vi "_builtins_rect_map_controls.vi"(11 "MasterBndRects in":T1[][](array[typedef])) -> (1 "row_heights":i16[](array[numeric]), 2 "column_widths":i16[](array[numeric]), 3 "Resolved MasterBndRects out":T1[][](array[typedef]))   [LabVIEW 2019, in "Script.lvlib"]
doc: "Resolves the front panel control bounds using a row and column mapper.\n\nCreated by: Ryan Pacini"
uses:
  Script.lvlib
  <vilib>/Utility/miscctls.llb/LVRectTypeDef.ctl
  <vilib>/Utility/miscctls.llb/LVBoundsTypeDef.ctl
  <vilib>/Utility/miscctls.llb/LVPositionTypeDef.ctl
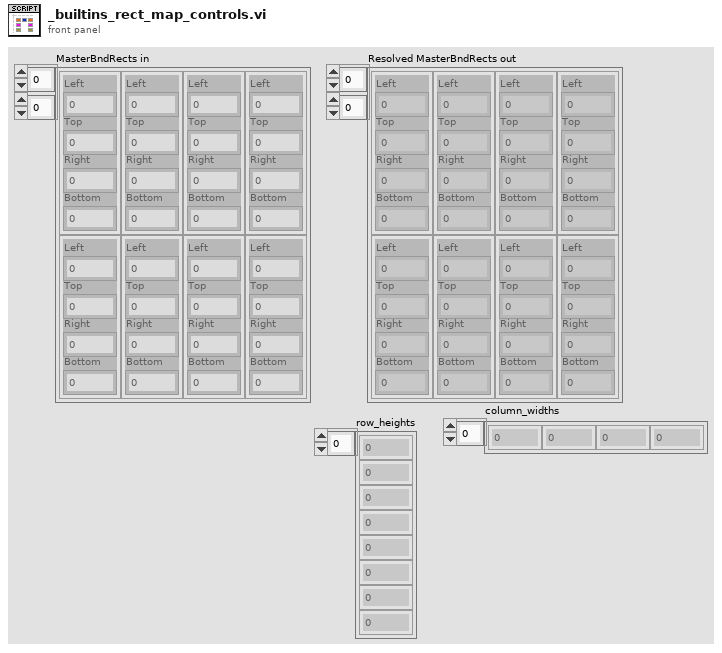
[diagram p1: front panel]
types:
  T1 = typedef "LVRectTypeDef.ctl" = cluster{"Left":i16, "Top":i16, "Right":i16, "Bottom":i16}
  T2 = typedef "LVBoundsTypeDef.ctl" = cluster{"Width":u32, "Height":u32}
  T3 = typedef "LVPositionTypeDef.ctl" = cluster{"Left":i32, "Top":i32}
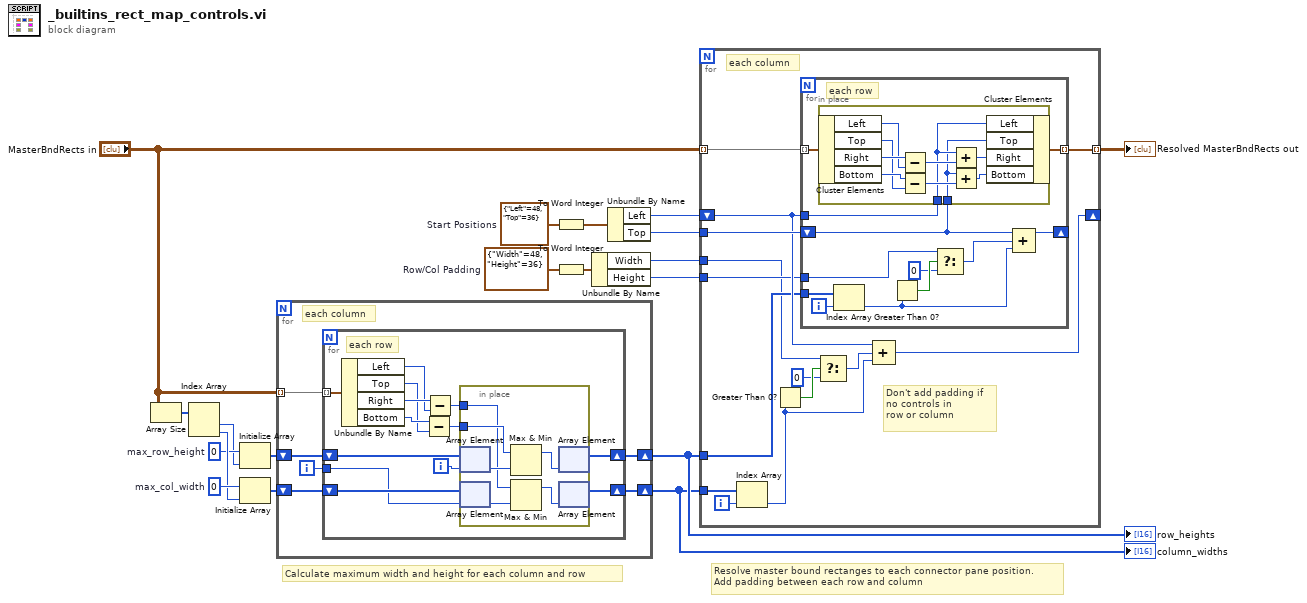
[diagram p0: block diagram]
diagram:
  w8 = i16 0  # max_row_height
  w12 = i16 0  # max_col_width
  w16 = T2 {"Width"=48, "Height"=36}  # Row/Col Padding
  w19 = T3 {"Left"=48, "Top"=36}  # Start Positions
  # "Resolve master bound rectanges to each connector pane position.\nAdd padding between each row and column"
  # "Calculate maximum width and height for each column and row"
  n1 = Array Size(array="MasterBndRects in") -> (size(s)=w11:i32[])
  n2 = Index Array(array=w11) -> (element #1=w7:i32, element #2=w9:i32)  [unwired: 2 in]
  n3 = Initialize Array(w8, w7) -> (w6:i16[])
  n4 = Initialize Array(w12, w9) -> (w4:i16[])
  n5 = for {
    tunnel: "MasterBndRects in" -> [w25] mode=indexing
    shift-right: [w23] -> w5
    shift-left: w6 -> [w24]
    shift-right: [w21] -> w3
    shift-left: w4 -> [w22]
    i -> [w20]
    # "each column"
    n6 = for {
      tunnel: w25 -> [w38] mode=indexing
      shift-right: [w29] -> w23
      shift-left: w24 -> [w33]
      shift-right: [w28] -> w21
      shift-left: w22 -> [w32]
      tunnel: w20 -> [w26]
      i -> [w27]
      # "each row"
      n7 = Unbundle By Name(w38) -> ("Left"=w35:i16, "Top"=w34:i16, "Right"=w37:i16, "Bottom"=w36:i16)
      n8 = Subtract(x=w36, y=w34) -> (x-y=w31:i16)
      n9 = Subtract(x=w37, y=w35) -> (x-y=w30:i16)
      n10 = in-place {
        in-place-border: w31 -> [w43]
        in-place-border: w30 -> [w40]
        n11 = in-place-array #1(w33, w27) -> (w44:i16)
        n12 = in-place-array #2(w32, w26) -> (w41:i16)
        n13 = Max & Min(x=w43, y=w44) -> (max(x,y)=w42:i16)  [unwired: 1 out]
        n14 = Max & Min(x=w40, y=w41) -> (max(x,y)=w39:i16)  [unwired: 1 out]
        n15 = in-place-array #1(w42) -> (w29:i16[])  [unwired: 1 out]
        n16 = in-place-array #2(w39) -> (w28:i16[])  [unwired: 1 out]
      }
    }
  }
  "row_heights" <- w5
  "column_widths" <- w3
  n17 = To Word Integer(number=w19) -> (16bit integer=w18:cluster{"Left":i16, "Top":i16})
  n18 = To Word Integer(number=w16) -> (16bit integer=w17:cluster{"Width":i16, "Height":i16})
  n19 = Unbundle By Name(w17) -> ("Width"=w2:i16, "Height"=w1:i16)
  n20 = Unbundle By Name(w18) -> ("Left"=w14:i16, "Top"=w13:i16)
  n21 = for {
    tunnel: "MasterBndRects in" -> [w57] mode=indexing
    tunnel: [w58] -> w15 mode=indexing
    tunnel: w5 -> [w52]
    shift-right: [w54] -> _
    shift-left: w14 -> [w55]
    tunnel: w13 -> [w56]
    tunnel: w3 -> [w51]
    tunnel: w2 -> [w46]
    tunnel: w1 -> [w50]
    i -> [w53]
    # "Don't add padding if\nno controls in\nrow or column"
    # "each column"
    n22 = Index Array(array=w51, index=w53) -> (element=w47:i16)
    n23 = Greater Than 0?(x=w47) -> (x > 0?=w49:bool)
    n24 = for {
      tunnel: [w70] -> w58 mode=indexing
      tunnel: w57 -> [w69] mode=indexing
      shift-right: [w68] -> _
      shift-left: w56 -> [w67]
      tunnel: w55 -> [w66]
      tunnel: w52 -> [w65]
      tunnel: w50 -> [w60]
      i -> [w64]
      # "each row"
      n25 = in-place {
        in-place-border: w67 -> [w71]
        in-place-border: w66 -> [w72]
        n26 = in-place-cluster #3(w69) -> ("Left"=w79:i16, "Top"=w77:i16, "Right"=w80:i16, "Bottom"=w78:i16)
        n27 = Subtract(x=w80, y=w79) -> (x-y=w76:i16)
        n28 = Subtract(x=w78, y=w77) -> (x-y=w74:i16)
        n29 = Add(x=w72, y=w76) -> (x+y=w75:i16)
        n30 = Add(x=w71, y=w74) -> (x+y=w73:i16)
        n31 = in-place-cluster #3("Left"=w72, "Top"=w71, "Right"=w75, "Bottom"=w73) -> (w70:T1)
      }
      n32 = Index Array(array=w65, index=w64) -> (element=w61:i16)
      n33 = Greater Than 0?(x=w61) -> (x > 0?=w63:bool)
      n34 = Select(t=w60, s=w63, f=i16 0) -> (s? t:f=w59:i16)
      n35 = Compound Arithmetic op=ADD(w67, w59, w61) -> (w68:i16)
    }
    n36 = Select(t=w46, s=w49, f=i16 0) -> (s? t:f=w48:i16)
    n37 = Compound Arithmetic op=ADD(w55, w48, w47) -> (w54:i16)
  }
  "Resolved MasterBndRects out" <- w15
